vi "Calibrate Ticks 2 Position (uSMC).vi"(1 "array index":i32, 2 "ticks":i32) -> (0 "value":dbl)   [LabVIEW 2010, in "SignalWriterMH110203USBStepperMotor.lvclass"]
uses:
  SignalWriterMH110203USBStepperMotor.lvclass
  class_data.vi
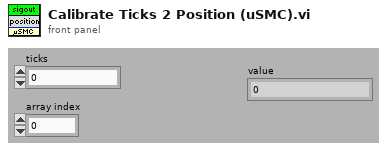
[diagram p1: front panel]
types:
  T1 = typedef "SignalWriterMH110203USBStepperMotor.lvclass/GoTo Control (uSMC).ctl" = cluster{"Step motor ID":string, "SMname":string, "Backlash":u16, "wait for input sygnal to start":bool, "use slow start/stop":bool, "units name":string, "Maximum speed":dbl, "speed":dbl, "step":u8, "point 1 ticks":i32, "point 2 ticks":i32, "point 1 units":dbl, "point 2 units":dbl, "Limit Switch standoff":dbl, "Zero Value":dbl, "Destination Position":dbl, "force backlash":bool, "power off when stop":bool, "POff delay":dbl, "positioner name":string, "R, Ohm":dbl, "I, mA":dbl, "Positioner's Type":u16, "Reset Direction":bool, "Manufacturer":string, "Model":string, "Scheme":string, "FirmwareVer":string}
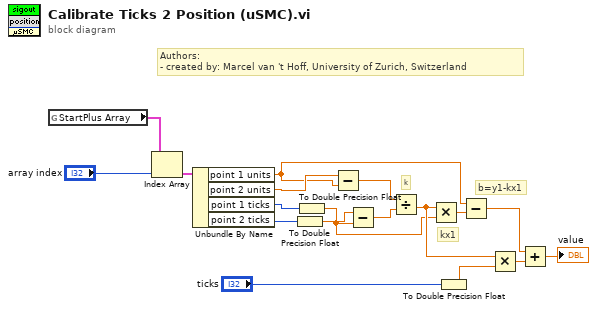
[diagram p0: block diagram]
diagram:
  # "Authors: \n- created by: Marcel van 't Hoff, University of Zurich, Switzerland"
  # "b=y1-kx1"
  # "kx1"
  # "k"
  n1 = global read "class_data.vi" "StartPlus Array"() -> (w16:T1[])
  n2 = Index Array(array=w16, index="array index") -> (element=w17:T1)
  n3 = Unbundle By Name(w17) -> ("point 1 units"=w1:dbl, "point 2 units"=w2:dbl, "point 1 ticks"=w5:i32, "point 2 ticks"=w4:i32)
  n4 = To Double Precision Float(number=w4) -> (double precision float=w11:dbl)
  n5 = To Double Precision Float(number=w5) -> (double precision float=w10:dbl)
  n6 = Subtract(x=w2, y=w1) -> (x-y=w7:dbl)
  n7 = Subtract(x=w11, y=w10) -> (x-y=w8:dbl)
  n8 = Divide(x=w7, y=w8) -> (x/y=w12:dbl)
  n9 = Multiply(x=w12, y=w10) -> (x*y=w9:dbl)
  n10 = To Double Precision Float(number="ticks") -> (double precision float=w13:dbl)
  n11 = Subtract(x=w1, y=w9) -> (x-y=w15:dbl)
  n12 = Multiply(x=w12, y=w13) -> (x*y=w14:dbl)
  n13 = Add(x=w15, y=w14) -> (x+y=→"value":dbl)
